vi "Read UI Console 1st CMD.vi"(8 "error in (no error)":errorcluster, 11 "UI Console MSG in":refnum<class "UI Console MSG.lvclass">) -> (0 "error out":errorcluster, 2 "UI Console 1st CMD":T1 caption="Enum 3", 3 "UI Console MSG out":refnum<class "UI Console MSG.lvclass">)   [LabVIEW 2024, in "UI Console MSG.lvclass"]
uses:
  UI Console MSG.lvclass
  Type Def/UI Console 1st CMD.ctl
  UI Console MSG.lvclass/UI Console MSG.ctl
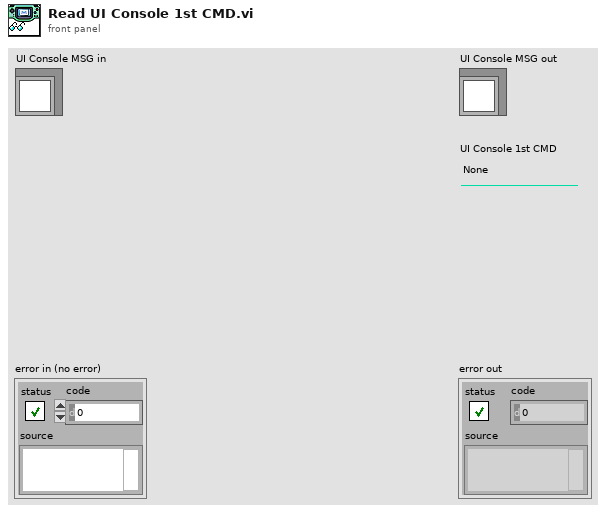
[diagram p1: front panel]
types:
  T1 = typedef "UI Console 1st CMD.ctl" = enum16{"None", "UI Manipulation", "UI Operation", "UI Stop"}
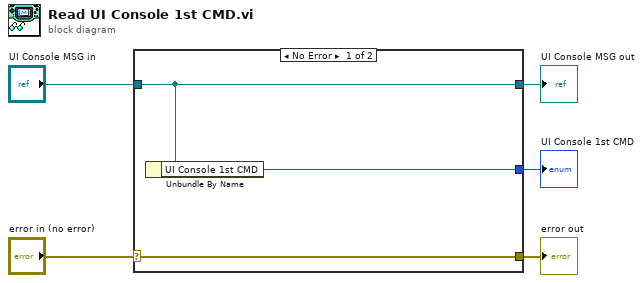
[diagram p0: block diagram]
diagram:
  n1 = case shown="No Error" "error in (no error)" {
    selector: "error in (no error)" -> [w8 w9]
    tunnel: [w8 w9] -> w4
    tunnel: [w7 w10] -> w2
    tunnel: "UI Console MSG in" -> [w7 w10]
    tunnel: [w6 _] -> w1
    frame No Error {
      n2 = Unbundle By Name(w7) -> ("UI Console 1st CMD"=w6:T1)
    }
    frame Error {
    }
  }
  "error out" <- w4
  "UI Console MSG out" <- w2
  "UI Console 1st CMD" <- w1
